vi "Test Parse setRefreshTime.vi"() -> ()   [LabVIEW 2019, in "Inst.Transport.lvclass"]
uses:
  Typedefs/RefreshTime--Request--Cluster.ctl
  25f8ba2b-0941-4ef6-b9d1-f01196d1bb40.vi
  25f8ba2b-0941-4ef6-b9d1-f01196d1bb40.vi/a641fe22-e98d-4282-89e8-e754ee14f500.vi
  25f8ba2b-0941-4ef6-b9d1-f01196d1bb40.vi/51551ffa-4ad3-4405-a8aa-0021968d8ddc.vi
  <vilib>/Utility/Data Type/Get Type Information.vi
  <vilib>/JDP Science/JSONtext/JSON text to Variant.vi
  <vilib>/JDP Science/JSONtext/LVClass Serializer/JSONtext LVClass Serializer.lvclass
  Inst.Transport.lvclass
  <vilib>/PRIrvin/JSON-RPC/JSON-RPC.lvlib
panel:
  out "Refresh Time 2":u32
  in  "Refresh Time":u32
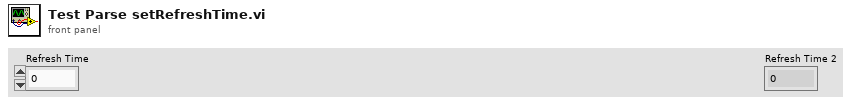
[diagram p1: front panel]
types:
  T1 = typedef "Inst.Transport.lvclass/RefreshTime--Request--Cluster.ctl" = cluster{"RefreshTime":u32}
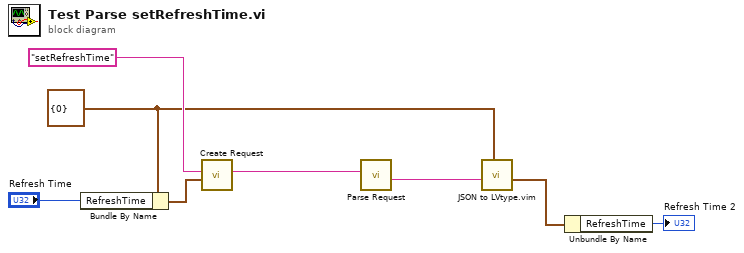
[diagram p0: block diagram]
diagram:
  w3 = T1 {"RefreshTime"=0} ("setRefreshTime")
  n1 = Bundle By Name(cluster=w3, "RefreshTime"="Refresh Time") -> (w8:T1)
  n2 = call <vilib>:"Create Request.vi"("params"=w8, "method"="setRefreshTime") -> ("<JSON> Requests"=w5:string)  [unwired: 7 in, 2 out]
  n3 = call <vilib>:"Parse Request.vi"("<JSON> Requests"=w5) -> ("Params"=w4:string)  [unwired: 7 in, 3 out]
  n4 = call "JSON to LVtype.vim"("type"=w3, "JSON Data in"=w4) -> ("Data out"=w2:T1)  [unwired: 8 in, 1 out]
  n5 = Unbundle By Name(w2) -> ("RefreshTime"=→"Refresh Time 2":u32)
